vi "USBImageContinuousV1.7.vi"() -> ()   [LabVIEW 2017]
uses:
  atmcd32d.dll
panel:
  in  "Tab Control":T1(tab)
  out "Expected position on spectrometer (pixels):":dbl
  in  "Harmonic":dbl min=10.0 max=40.0
  out "l (nm)":dbl
  out "E (J)":dbl
  out "E (eV)":dbl
  out "Nearest Harmonic of 800nm":dbl
  out "Cursor Position (pixels)":dbl
  out "Distance to nearest harmonic of 800nm (pixels)":dbl
  in  "Grating:":u16(ring) items=["Shimadzu 30-006  "]
  in  "Laser:":u16(ring) items=["800nm  "]
  in  "Trigger":u32(ring) items=["Internal", "External"]
  in  "Exposure Time (secs)":sgl format="%.2f"
  out "Get Acquired Data":u32
  out "Start Acquisition":u32
  out "Detector X Pixels":i32
  out "Detector Y Pixels":i32
  out "Shut Down":u32
  out "Raw Image":i32[][](graph)
  out "Vertical Binned image":i32[](graph)
  out "Get Status":u32
  in  "Stop":bool
  in  "Save Image":bool
  out "Camera Status:":bool
  out "Last Image Saved:":string
  in  "Calibration Date":u16(ring) items=["first calibration - 7/31", "7/31-current"]
  out "Calibration Date: indicator:":u16(ring) items=["first calibration - 7/31", "7/31-current"]
  out "Status":u32
  out "Camera outputs":T2
  out "Camera inputs":T3
  out "Wavelength Graph (nm)":cluster{"No prefix":dbl, i32}[](graph)
  out "Energy Graph (eV)":cluster{"eV":dbl, i32}[](graph)
  out "Harmonics Graph":cluster{"No prefix":dbl, i32}[](graph)
  # "Acquisition Mode: Single Scan\nReadout Mode: Full Resolution Image"
  # "Return values"
  # "XUV Spectrometer Control VI"
  # "Status"
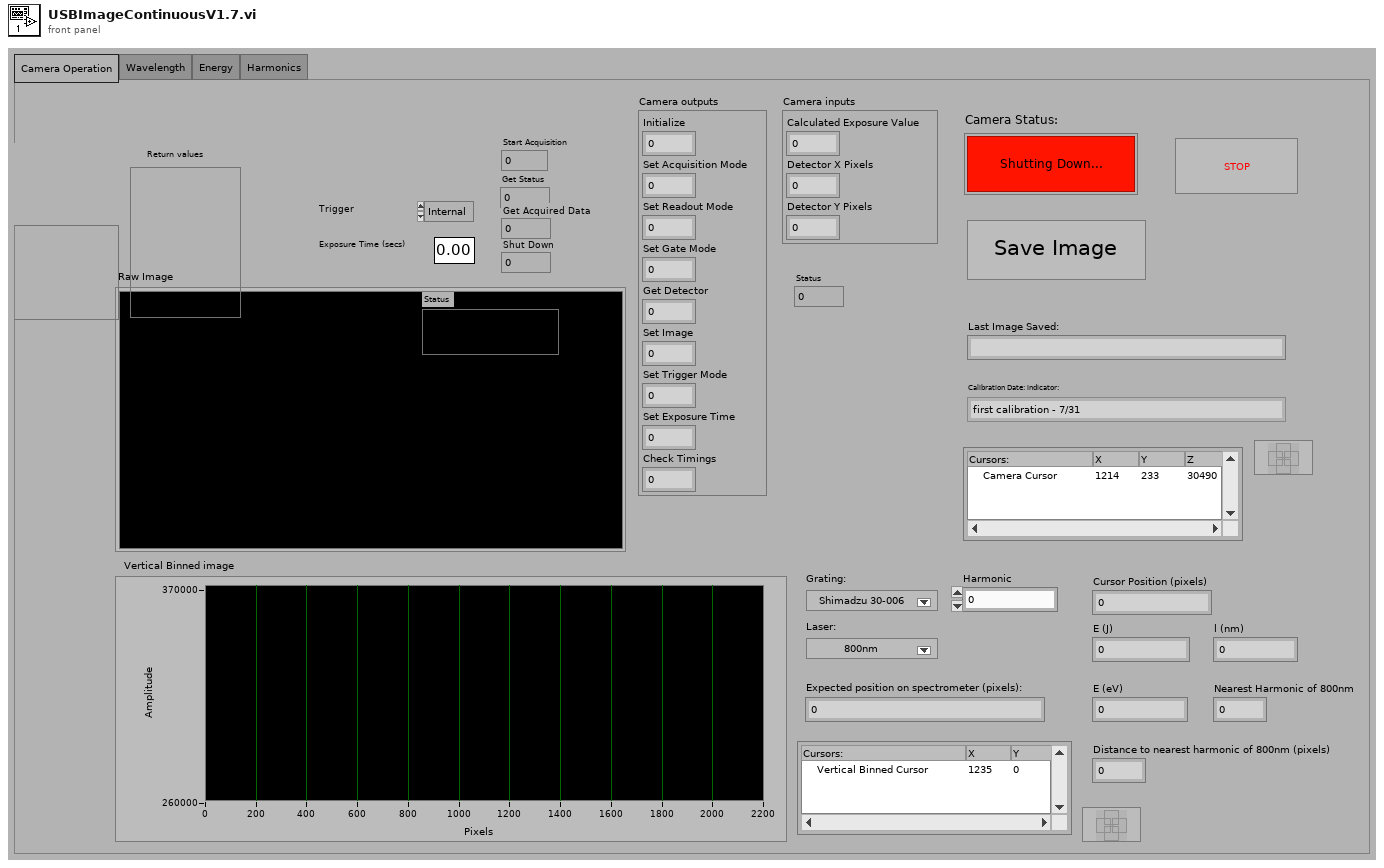
[diagram p1: front panel]
types:
  T1 = enum32{"Camera Operation", "Wavelength", "Energy", "Harmonics"}
  T2 = cluster{"Initialize":u32, "Set Acquisition Mode":u32, "Set Readout Mode":u32, "Set Gate Mode":u32, "Get Detector":u32, "Set Image":u32, "Set Trigger Mode":u32, "Set Exposure Time":u32, "Check Timings":u32}
  T3 = cluster{"Calculated Exposure Value":sgl, "Detector X Pixels":i32, "Detector Y Pixels":i32}
  T4 = cluster{"to shutdown":bool, "to get acquired data":bool, "to start acquisition":bool, "DRV_SUCCESS":i32}
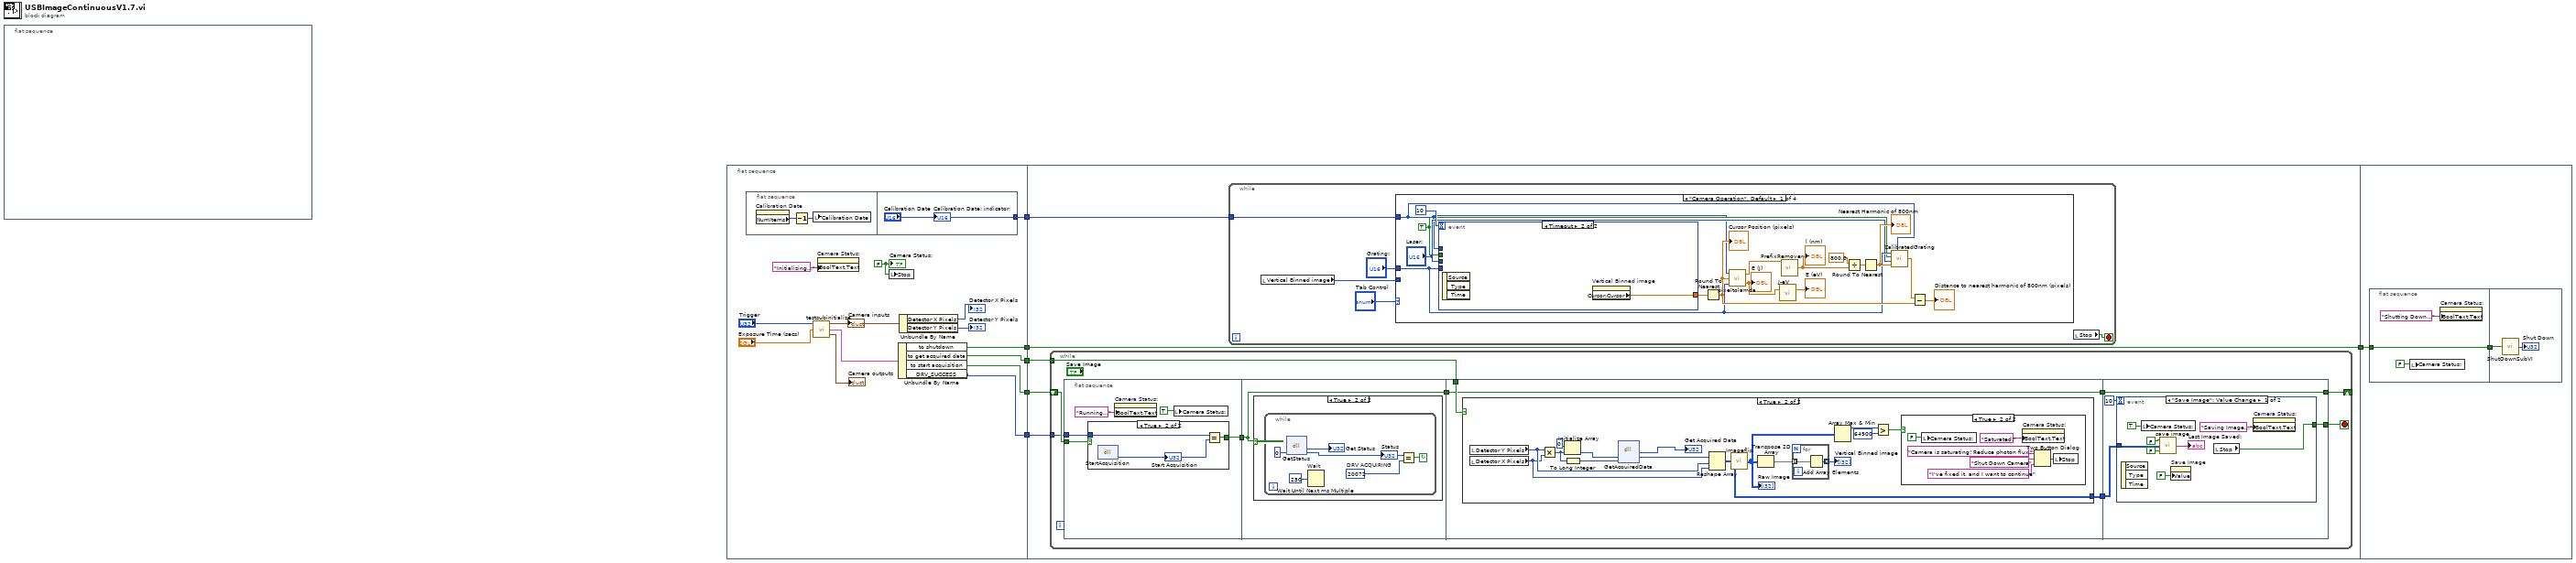
[diagram p0: block diagram]
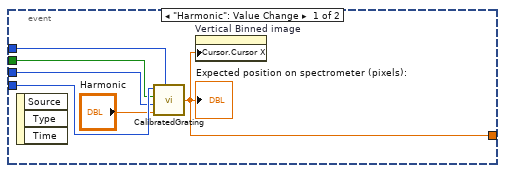
[diagram p2: hidden frame]
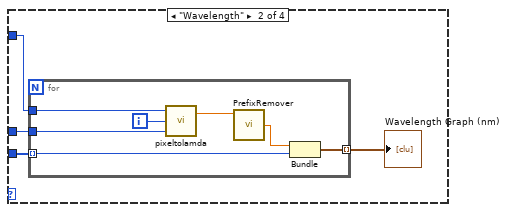
[diagram p3: hidden frame]
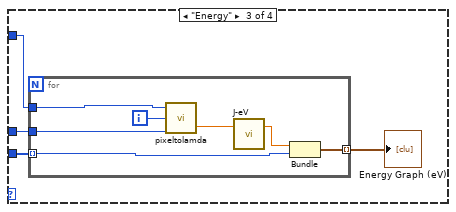
[diagram p4: hidden frame]
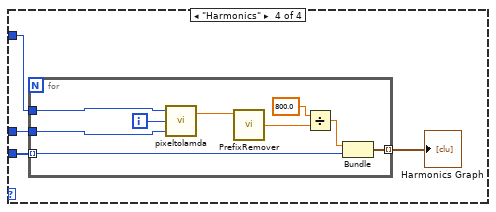
[diagram p5: hidden frame]
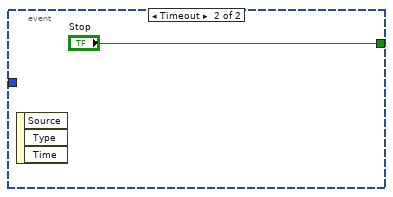
[diagram p10: hidden frame]
diagram:
  n1 = flat-sequence {
    frame #0 {
    }
  }
  n2 = flat-sequence {
    tunnel: [w7] -> w5
    tunnel: [w8] -> w4
    tunnel: [w9] -> w3
    tunnel: [w10] -> w2
    tunnel: [w20] -> w1
    tunnel: [w25] -> w6
    tunnel: w5 -> [w28]
    tunnel: w4 -> [w27]
    tunnel: w3 -> [w26]
    tunnel: w2 -> [w25]
    tunnel: w1 -> [w24]
    tunnel: w6 -> [w156]
    frame #0 {
      w19 = FALSE ("Camera Status:")
      n3 = flat-sequence {
        tunnel: ["Calibration Date"] -> w20
        frame #0 {
          n4 = property on="Calibration Date" class="Ring (strict)"() -> ("NumItems"=w22:u32)  [unwired: 2 in, 2 out]
          n5 = Decrement(x=w22) -> (x-1=w21:u32)
          n6 = local write "Calibration Date"(w21) -> ()
        }
        frame #1 {
          "Calibration Date: indicator:" <- "Calibration Date"
        }
      }
      n7 = call "testsubinitialize.vi"("Exposure Time (secs)"="Exposure Time (secs)", "Trigger"="Trigger") -> ("Camera outputs"=→"Camera outputs":T2, "Camera status"=w17:T4, "Camera inputs"=w14:T3)  [unwired: 1 in]
      "Camera inputs" <- w14
      n8 = property on="Camera Status:" class="Bool (strict)"("BoolText.Text"="Initializing..." ("String")) -> ()  [unwired: 2 in, 2 out]
      n9 = local write "Stop"(w19) -> ()
      n10 = Unbundle By Name(w17) -> ("to shutdown"=w10:bool, "to get acquired data"=w9:bool, "to start acquisition"=w8:bool, "DRV_SUCCESS"=w7:i32)
      n11 = Unbundle By Name(w14) -> ("Detector X Pixels"=→"Detector X Pixels":i32, "Detector Y Pixels"=→"Detector Y Pixels":i32)
      "Camera Status:" <- w19
    }
    frame #1 {
      n12 = while {
        tunnel: w28 -> [w99]
        tunnel: w26 -> [w98]
        shift-right: [w94] -> _
        shift-left: w27 -> [w100]
        stop <- w92 stop-if-true
        n13 = flat-sequence {
          tunnel: w100 -> [w105]
          tunnel: w99 -> [w104]
          tunnel: [w103] -> w97
          tunnel: w97 -> [w110]
          tunnel: [w110] -> w96
          tunnel: w96 -> [w118]
          tunnel: w98 -> [w119]
          tunnel: [w118] -> w95
          tunnel: [w117] -> w93
          tunnel: w95 -> [w146]
          tunnel: w93 -> [w143]
          tunnel: [w144] -> w92
          tunnel: [w146] -> w94
          frame #0 {
            n14 = case shown="True" w105 {
              tunnel: [FALSE w109] -> w103
              tunnel: w104 -> [_ w108]
              frame False {
              }
              frame True {
                n15 = dll-call lib="atmcd32d.dll" fn="StartAcquisition" label="Call Library Function start acquisition"() -> (w107:u32)  [unwired: 3 in, 2 out]
                "Start Acquisition" <- w107
                n16 = Equal?(x=w108, y=w107) -> (x = y?=w109:bool)
              }
            }
            n17 = property on="Camera Status:" class="Bool (strict)"("BoolText.Text"="Running..." ("Boolean Text.Text")) -> ()  [unwired: 2 in, 2 out]
            n18 = local write "Camera Status:"(TRUE ("Camera Status:")) -> ()
          }
          frame #1 {
            n19 = case shown="True" w110 {
              frame False {
              }
              frame True {
                n20 = while {
                  stop <- w114 continue-if-true
                  w113 = u16 20072  # DRV ACQUIRING
                  n21 = dll-call lib="atmcd32d.dll" fn="GetStatus" label="Call Library Function GetAcquisitionStatus"(u16 0) -> (→"Get Status":u32, w112:u32)  [unwired: 3 in, 2 out]
                  "Status" <- w112
                  n22 = Wait Until Next ms Multiple "Wait"(millisecond multiple=u32 250) -> ()  [unwired: 1 out]
                  n23 = Equal?(x=w112, y=w113) -> (x = y?=w114:bool)
                }
              }
            }
          }
          frame #2 {
            n24 = case shown="True" w119 {
              tunnel: [_ w123] -> w117
              frame False {
              }
              frame True {
                n25 = local read "Detector Y Pixels"() -> (w129:i32)
                n26 = local read "Detector X Pixels"() -> (w125:i32)
                n27 = Multiply(x=w129, y=w125) -> (x*y=w131:i32)
                n28 = Initialize Array "Initialize Array"(0 ("Initial values in array"), w131) -> (w133:i32[])
                n29 = To Long Integer(number=w131) -> (32bit integer=w132:i32)
                n30 = dll-call lib="atmcd32d.dll" fn="GetAcquiredData" label="Call Library Function Get Acquired data"(w133, w132) -> (→"Get Acquired Data":u32, w130:i32[])  [unwired: 4 in, 2 out]
                n31 = Reshape Array(w130, w129, w125) -> (w123:i32[][])
                n32 = call "Imageflip.vi"("2D array"=w123) -> ("transposed array"=w121:i32[][])
                "Raw Image" <- w121
                n33 = Transpose 2D Array(2D array=w121) -> (transposed array=w128:i32[][])
                n34 = for {
                  tunnel: w128 -> [w142] mode=indexing
                  tunnel: [w141] -> w122 mode=indexing
                  n35 = Add Array Elements(numeric array=w142) -> (sum=w141:i32)
                }
                "Vertical Binned image" <- w122
                n36 = Array Max & Min(array=w121) -> (max value=w127:i32)  [unwired: 3 out]
                n37 = Greater?(x=w127, y=64900) -> (0:w126:bool)
                n38 = case shown="True" w126 {
                  frame False {
                  }
                  frame True {
                    n39 = local write "Camera Status:"(FALSE ("Camera Status:")) -> ()
                    n40 = property on="Camera Status:" class="Bool (strict)"("BoolText.Text"="Saturated!" ("Boolean Text.Text")) -> ()  [unwired: 2 in, 2 out]
                    n41 = Two Button Dialog(message="Camera is saturating! Reduce photon flux!", 1:"I've fixed it, and I want to continue" ("message"), 2:"Shut Down Camera" ("T button name (\"OK\")")) -> (T button?=w136:bool)
                    n42 = local write "Stop"(w136) -> ()
                  }
                }
              }
            }
          }
          frame #3 {
            n43 = event shown="[0] \"Save Image\": Value Change" {
              selector: _ -> [_ _]
              dyn-events: _ -> [_ _]
              timeout: 10 -> [_ _]
              tunnel: [w151 "Stop"] -> w144
              tunnel: w143 -> [w150 _]
              event "Save Image": Value Change {
                n44 = event-data() -> ()  [unwired: 1 in, 3 out]
                n45 = local write "Camera Status:"(TRUE ("Camera Status:")) -> ()
                n46 = call "save image.vi"("Start of pump/prove run?"=FALSE, "Image to save"=w150, "Pump/probe run?"=FALSE) -> ("Image file path"=→"Last Image Saved:":string)
                n47 = property on="Save Image" class="Bool (strict)"("Value"=FALSE ("Take image")) -> ()  [unwired: 2 in, 2 out]
                n48 = local read "Stop"() -> (w151:bool)
                n49 = property on="Camera Status:" class="Bool (strict)"("BoolText.Text"="Saving Image..." ("Boolean Text.Text")) -> ()  [unwired: 2 in, 2 out]
              }
              event Timeout {
                n50 = event-data() -> ()  [unwired: 1 in, 3 out]
              }
            }
          }
        }
      }
      n51 = while {
        tunnel: w24 -> [w29]
        stop <- w30 stop-if-true
        n52 = local read "Vertical Binned image"() -> (w32:i32[])
        n53 = case shown="\"Camera Operation\", Default" "Tab Control" {
          tunnel: w32 -> [_ w60 w71 w82]
          tunnel: "Grating:" -> [w37 w59 w70 w81]
          tunnel: w29 -> [w34 w57 w68 w79]
          frame "Camera Operation", Default {
            w36 = TRUE
            n54 = event shown="[1] Timeout" {
              selector: _ -> [_ _]
              dyn-events: _ -> [_ _]
              timeout: 10 -> [_ _]
              tunnel: [w51 w56] -> w38
              tunnel: w37 -> [w55 _]
              tunnel: w36 -> [w54 _]
              tunnel: "Laser:" -> [w53 _]
              tunnel: w34 -> [w52 _]
              event "Harmonic": Value Change {
                n55 = event-data() -> ()  [unwired: 1 in, 3 out]
                n56 = call "CalibratedGrating.vi"("Grating:"=w55, "Subvi?"=w54, "Laser:"=w53, "Harmonic"="Harmonic", "Caibration Date"=w52) -> ("Position on spectrometer (pixels):"=w51:dbl)
                "Expected position on spectrometer (pixels):" <- w51
                n57 = property on="Vertical Binned image" class="WFGraph (strict)"("Cursor.Cursor X"=w51) -> ()  [unwired: 2 in, 2 out]
              }
              event Timeout {
                n58 = event-data() -> ()  [unwired: 1 in, 3 out]
                n59 = property on="Vertical Binned image" class="WFGraph (strict)"() -> ("Cursor.Cursor X"=w56:dbl)  [unwired: 2 in, 2 out]
              }
            }
            n60 = Round To Nearest(number=w38) -> (nearest integer value=w43:dbl)
            "Cursor Position (pixels)" <- w43
            n61 = call "pixeltolamda.vi"("Grating:"=w37, "Pixel Postion"=w43, "Caibration Date"=w34) -> ("E (J)"=w45:dbl, "lamda (m)"=w49:dbl)
            "E (J)" <- w45
            n62 = call "J-eV.vi"("J"=w45) -> ("eV"=→"E (eV)":dbl)  [unwired: 1 in, 1 out]
            n63 = call "PrefixRemover.vi"("Nano"=w49) -> ("No prefix"=w46:dbl)  [unwired: 3 in]
            "l (nm)" <- w46
            n64 = Divide(x=800.0, y=w46) -> (x/y=w48:dbl)
            n65 = Round To Nearest(number=w48) -> (nearest integer value=w42:dbl)
            "Nearest Harmonic of 800nm" <- w42
            n66 = call "CalibratedGrating.vi"("Grating:"=w37, "Subvi?"=w36, "Laser:"="Laser:", "Harmonic"=w42, "Caibration Date"=w34) -> ("Position on spectrometer (pixels):"=w41:dbl)
            n67 = Subtract(x=w41, y=w43) -> (x-y=→"Distance to nearest harmonic of 800nm (pixels)":dbl)
          }
          frame "Wavelength" {
            n68 = for {
              tunnel: w60 -> [w63] mode=indexing
              tunnel: w59 -> [w65]
              tunnel: [w62] -> w58 mode=indexing
              tunnel: w57 -> [w61]
              i -> [w64]
              n69 = call "pixeltolamda.vi"("Grating:"=w65, "Pixel Postion"=w64, "Caibration Date"=w61) -> ("lamda (m)"=w66:dbl)  [unwired: 1 out]
              n70 = call "PrefixRemover.vi"("Nano"=w66) -> ("No prefix"=w67:dbl)  [unwired: 3 in]
              n71 = Bundle("No prefix"=w67, w63) -> (w62:cluster{"No prefix":dbl, i32})  [unwired: 1 in]
            }
            "Wavelength Graph (nm)" <- w58
          }
          frame "Energy" {
            n72 = for {
              tunnel: w71 -> [w74] mode=indexing
              tunnel: w70 -> [w77]
              tunnel: [w73] -> w69 mode=indexing
              tunnel: w68 -> [w72]
              i -> [w78]
              n73 = call "pixeltolamda.vi"("Grating:"=w77, "Pixel Postion"=w78, "Caibration Date"=w72) -> ("E (J)"=w76:dbl)  [unwired: 1 out]
              n74 = call "J-eV.vi"("J"=w76) -> ("eV"=w75:dbl)  [unwired: 1 in, 1 out]
              n75 = Bundle("eV"=w75, w74) -> (w73:cluster{"eV":dbl, i32})  [unwired: 1 in]
            }
            "Energy Graph (eV)" <- w69
          }
          frame "Harmonics" {
            n76 = for {
              tunnel: w82 -> [w88] mode=indexing
              tunnel: w81 -> [w90]
              tunnel: [w87] -> w80 mode=indexing
              tunnel: w79 -> [w83]
              i -> [w89]
              n77 = call "pixeltolamda.vi"("Grating:"=w90, "Pixel Postion"=w89, "Caibration Date"=w83) -> ("lamda (m)"=w91:dbl)  [unwired: 1 out]
              n78 = call "PrefixRemover.vi"("Nano"=w91) -> ("No prefix"=w85:dbl)  [unwired: 3 in]
              n79 = Divide(x=800.0, y=w85) -> (x/y=w84:dbl)
              n80 = Bundle(w84, w88) -> (w87:cluster{dbl, i32})  [unwired: 1 in]
            }
            "Harmonics Graph" <- w80
          }
        }
        n81 = local read "Stop"() -> (w30:bool)
      }
    }
    frame #2 {
      n82 = flat-sequence {
        tunnel: w156 -> [w160]
        tunnel: [w160] -> w157
        tunnel: w157 -> [w162]
        frame #0 {
          n83 = local write "Camera Status:"(FALSE ("Camera Status:")) -> ()
          n84 = property on="Camera Status:" class="Bool (strict)"("BoolText.Text"="Shutting Down..." ("Boolean Text.Text")) -> ()  [unwired: 2 in, 2 out]
        }
        frame #1 {
          n85 = call "ShutDownSubVI.vi"("shutdown"=w162) -> ("Shut Down"=→"Shut Down":u32)
        }
      }
    }
  }
